vi "SR830_Manage_Monitor.vi"(3 "Lockin # (in)":i32, 4 "System Monitor Variables (in)":T1, 5 "Global Status (in)":T2={"Lockin 1"=[], "X1-Display"=0.0, "Y1-Display"=0.0, "X1 Percent"=0.0, "X1 Overload"=FALSE, "Y1 Overload"=FALSE, "Unit X1"="nV", "Unit X2"="nV", "Unit X2a"="nV", "Unit X1a"="nV", "Sensitivity Setpoint"=26, "X1 Percent 2"=0.0, "Y1"=0.0, "X1"=0.0, "Preamp OVL"=FALSE} {"X1 Percent 2" scale=0.0..1.0; "Sensitivity Setpoint" items=["2 nV", "5 nV", "10 nV", "20 nV", "50 nV", "100 nV", "200 nV", "500 nV", "1 µV", "2 µV", "5 µV", "10 µV", "20 µV", "50 µV", "100 µV", "200 µV", "500 µV", "1 mV", "2 mV", "5 mV", "10 mV", "20 mV", "50 mV", "100 mV", "200 mV", "500 mV", "1 V", ""]; "X1 Percent" scale=0.0..1.0; "X1-Display" format="%#4_5f"}, 6 "Command (in)":T2={"Lockin 1"=[], "X1-Display"=0.0, "Y1-Display"=0.0, "X1 Percent"=0.0, "X1 Overload"=FALSE, "Y1 Overload"=FALSE, "Unit X1"="nV", "Unit X2"="nV", "Unit X2a"="nV", "Unit X1a"="nV", "Sensitivity Setpoint"=26, "X1 Percent 2"=0.0, "Y1"=0.0, "X1"=0.0, "Preamp OVL"=FALSE} {"X1 Percent 2" scale=0.0..1.0; "Sensitivity Setpoint" items=["2 nV", "5 nV", "10 nV", "20 nV", "50 nV", "100 nV", "200 nV", "500 nV", "1 µV", "2 µV", "5 µV", "10 µV", "20 µV", "50 µV", "100 µV", "200 µV", "500 µV", "1 mV", "2 mV", "5 mV", "10 mV", "20 mV", "50 mV", "100 mV", "200 mV", "500 mV", "1 V", ""]; "X1 Percent" scale=0.0..1.0; "X1-Display" format="%#4_5f"}, 7 "queue (in)":refnum<queue>) -> (0 "System Monitor Variables (out)":T1, 1 "Monitor (out)":T2={"Lockin 1"=[], "X1-Display"=0.0, "Y1-Display"=0.0, "X1 Percent"=0.0, "X1 Overload"=FALSE, "Y1 Overload"=FALSE, "Unit X1"="nV", "Unit X2"="nV", "Unit X2a"="nV", "Unit X1a"="nV", "Sensitivity Setpoint"=26, "X1 Percent 2"=0.0, "Y1"=0.0, "X1"=0.0, "Preamp OVL"=FALSE} {"X1 Percent 2" scale=0.0..1.0; "Sensitivity Setpoint" items=["2 nV", "5 nV", "10 nV", "20 nV", "50 nV", "100 nV", "200 nV", "500 nV", "1 µV", "2 µV", "5 µV", "10 µV", "20 µV", "50 µV", "100 µV", "200 µV", "500 µV", "1 mV", "2 mV", "5 mV", "10 mV", "20 mV", "50 mV", "100 mV", "200 mV", "500 mV", "1 V", ""]; "X1 Percent" scale=0.0..1.0; "X1-Display" format="%#4_5f"})   [LabVIEW 2019]
uses:
  SR830/SR830-Cluster.ctl
  Global/Global Variables/System Monitor Cluster.ctl
  Instrument_Setup.vi
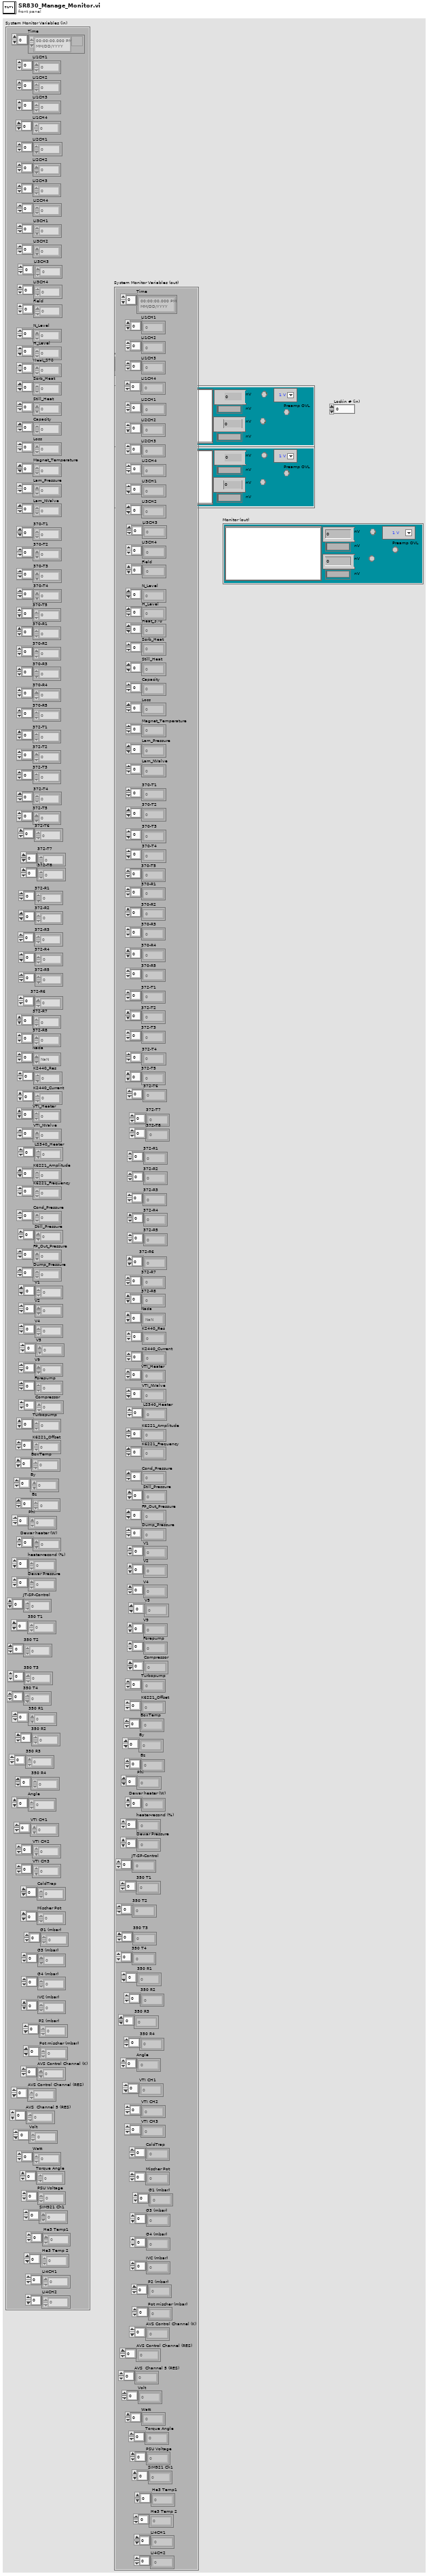
[diagram p1: front panel]
types:
  T1 = typedef "System Monitor Cluster.ctl" = cluster{"Time":timestamp[], "LI1CH1":dbl[], "LI1CH2":dbl[], "LI2CH1":dbl[], "LI2CH2":dbl[], "LI3CH1":dbl[], "LI3CH2":dbl[], "Field":dbl[], "N_Level":dbl[], "H_Level":dbl[], "Heat_370":dbl[], "Sorb_Heat":dbl[], "Still_Heat":dbl[], "Capacity":dbl[], "Loss":dbl[], "Magnet_Temperature":dbl[], "Lam_Pressure":dbl[], "Lam_NValve":dbl[], "370-T1":dbl[], "370-T2":dbl[], "370-T3":dbl[], "370-T4":dbl[], "370-T5":dbl[], "370-R1":dbl[], "370-R2":dbl[], "370-R3":dbl[], "370-R4":dbl[], "370-R5":dbl[], "372-T1":dbl[], "372-T2":dbl[], "372-T3":dbl[], "372-T4":dbl[], "372-T5":dbl[], "372-T6":dbl[], "372-R1":dbl[], "372-R2":dbl[], "372-R3":dbl[], "372-R4":dbl[], "372-R5":dbl[], "372-R6":dbl[], "Nada":dbl[], "K2440_Res":dbl[], "K2440_Current":dbl[], "VTI_Heater":dbl[], "VTI_NValve":dbl[], "LS340_Heater":dbl[], "K6221_Amplitude":dbl[], "K6221_Frequency":dbl[], "Cond_Pressure":dbl[], "Still_Pressure":dbl[], "FP_Out_Pressure":dbl[], "Dump_Pressure":dbl[], "V1":dbl[], "V2":dbl[], "V4":dbl[], "V5":dbl[], "V9":dbl[], "Forepump":dbl[], "Compressor":dbl[], "K6221_Offset":dbl[], "BoxTemp":dbl[], "By":dbl[], "Bz":dbl[], "Phi":dbl[], "heater-recond (%)":dbl[], "Dewar Pressure ":dbl[], "JT-SP-Control":dbl[], "350 T1":dbl[], "350 T2":dbl[], "350 T3":dbl[], "350 T4":dbl[], "350 R1":dbl[], "350 R2":dbl[], "350 R3":dbl[], "350 R4":dbl[], "Angle":dbl[], "VTI CH1":dbl[], "VTI CH2":dbl[], "VTI CH3":dbl[], "ColdTrap":dbl[], "Mischer Pot":dbl[], "G1 (mbar)":dbl[], "G3 (mbar) ":dbl[], "G4 (mbar)":dbl[], "IVC (mbar)":dbl[], "P2 (mbar) ":dbl[], "Pot mischer (mbar)":dbl[], "AVS Control Channel (K)":dbl[], "AVS Control Channel (RES)":dbl[], "AVS  Channel 5 (RES) ":dbl[], "LI3CH3":dbl[], "LI3CH4":dbl[], "LI1CH3":dbl[], "LI1CH4":dbl[], "LI2CH3":dbl[], "LI2CH4":dbl[], "Volt":dbl[], "Watt":dbl[], "Torque Angle":dbl[], "Dewar heater (W)":dbl[], "PSU Voltage":dbl[], "Turbopump":dbl[], "372-R7":dbl[], "372-T7":dbl[], "SIM921 Ch1":dbl[], " He3 Temp1":dbl[], " He3 Temp 2":dbl[], "LI4CH1":dbl[], "LI4CH2":dbl[], "372-T8":dbl[], "372-R8":dbl[]}
  T2 = typedef "SR830-Cluster.ctl" = cluster{"Lockin 1":dbl[][], "X1-Display":dbl, "Y1-Display":dbl, "X1 Percent":dbl, "X1 Overload":bool, "Y1 Overload":bool, "Unit X1":string, "Unit X2":string, "Unit X2a":string, "Unit X1a":string, "Sensitivity Setpoint":i16, "X1 Percent 2":dbl, "Y1":dbl, "X1":dbl, "Preamp OVL":bool}
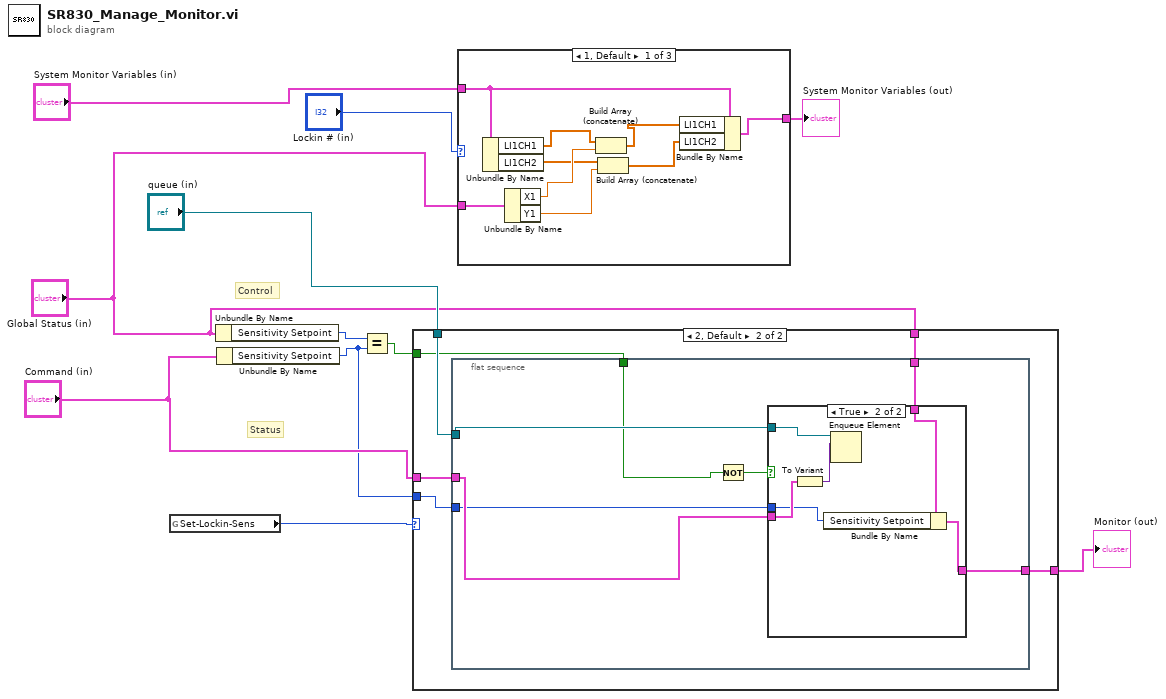
[diagram p0: block diagram]
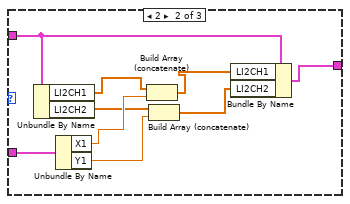
[diagram p4: hidden frame]
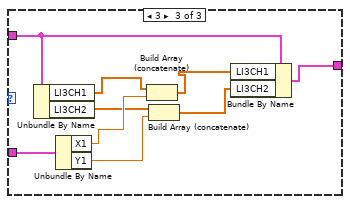
[diagram p5: hidden frame]
diagram:
  # "Status"
  # "Control"
  n1 = global read "Instrument_Setup.vi" "Set-Lockin-Sens"() -> (w1:u16)
  n2 = Unbundle By Name("Global Status (in)") -> ("Sensitivity Setpoint"=w3:i16)
  n3 = Unbundle By Name("Command (in)") -> ("Sensitivity Setpoint"=w2:i16)
  n4 = Equal?(x=w3, y=w2) -> (x = y?=w10:bool)
  n5 = case shown="2, Default" w1 {
    tunnel: "queue (in)" -> [_ w18]
    tunnel: w10 -> [_ w17]
    tunnel: [w12 w16] -> w9
    tunnel: "Command (in)" -> [_ w15]
    tunnel: "Global Status (in)" -> [w12 w14]
    tunnel: w2 -> [_ w13]
    frame 0, 1 {
    }
    frame 2, Default {
      n6 = flat-sequence {
        tunnel: w18 -> [w25]
        tunnel: w15 -> [w22]
        tunnel: [w23] -> w16
        tunnel: w17 -> [w21]
        tunnel: w14 -> [w20]
        tunnel: w13 -> [w19]
        frame #0 {
          n7 = Not(x=w21) -> (.not. x?=w24:bool)
          n8 = case shown="True" w24 {
            tunnel: w25 -> [_ w32]
            tunnel: w22 -> [_ w30]
            tunnel: [w26 w27] -> w23
            tunnel: w20 -> [w26 w29]
            tunnel: w19 -> [_ w28]
            frame False {
            }
            frame True {
              n9 = To Variant(anything=w30) -> (Variant=w31:variant)
              n10 = Bundle By Name(cluster=w29, "Sensitivity Setpoint"=w28) -> (w27:T2)
              n11 = Enqueue Element(queue=w32, element=w31) -> ()  [unwired: 2 in, 3 out]
            }
          }
        }
      }
    }
  }
  "Monitor (out)" <- w9
  n12 = case shown="1, Default" "Lockin # (in)" {
    tunnel: "Global Status (in)" -> [w41 w50 w59]
    tunnel: "System Monitor Variables (in)" -> [w40 w49 w58]
    tunnel: [w33 w42 w51] -> w5
    frame 1, Default {
      n13 = Unbundle By Name(w40) -> ("LI1CH1"=w38:dbl[], "LI1CH2"=w36:dbl[])
      n14 = Unbundle By Name(w41) -> ("X1"=w39:dbl, "Y1"=w35:dbl)
      n15 = Build Array (concatenate)(w38, w39) -> (w37:dbl[])
      n16 = Build Array (concatenate)(w36, w35) -> (w34:dbl[])
      n17 = Bundle By Name(cluster=w40, "LI1CH1"=w37, "LI1CH2"=w34) -> (w33:T1)
    }
    frame 2 {
      n18 = Unbundle By Name(w49) -> ("LI2CH1"=w47:dbl[], "LI2CH2"=w45:dbl[])
      n19 = Unbundle By Name(w50) -> ("X1"=w48:dbl, "Y1"=w44:dbl)
      n20 = Build Array (concatenate)(w47, w48) -> (w46:dbl[])
      n21 = Build Array (concatenate)(w45, w44) -> (w43:dbl[])
      n22 = Bundle By Name(cluster=w49, "LI2CH1"=w46, "LI2CH2"=w43) -> (w42:T1)
    }
    frame 3 {
      n23 = Unbundle By Name(w58) -> ("LI3CH1"=w56:dbl[], "LI3CH2"=w54:dbl[])
      n24 = Unbundle By Name(w59) -> ("X1"=w57:dbl, "Y1"=w53:dbl)
      n25 = Build Array (concatenate)(w56, w57) -> (w55:dbl[])
      n26 = Build Array (concatenate)(w54, w53) -> (w52:dbl[])
      n27 = Bundle By Name(cluster=w58, "LI3CH1"=w55, "LI3CH2"=w52) -> (w51:T1)
    }
  }
  "System Monitor Variables (out)" <- w5
